vi "Configure Output Impedance.vi"(8 "error in (no error)":errorcluster, 10 "Impedance (0: 50 Ohms)":u16(ring) items=["50 Ohms", "High Impedance"], 11 "VISA resource name":refnum<visa-resource-name>) -> (0 "error out":errorcluster, 3 "VISA resource name out":refnum<visa-resource-name>)   [LabVIEW 2015, in "Template - Function Generator.lvlib"]
doc: "Configures the output impedance for the function generator."
uses:
  <instrlib>/_Template - Function Generator/Template - Function Generator.lvlib
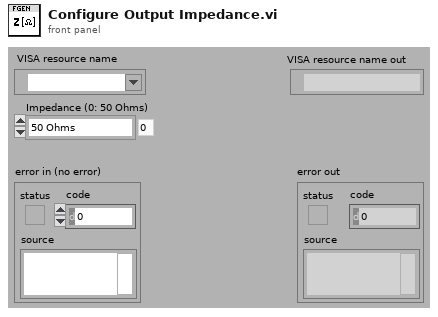
[diagram p1: front panel]
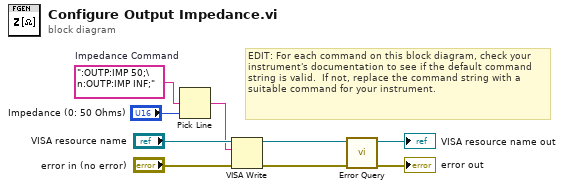
[diagram p0: block diagram]
diagram:
  w3 = ":OUTP:IMP 50;\n:OUTP:IMP INF;"  # Impedance Command
  # "EDIT: For each command on this block diagram, check your instrument's documentation to see if the default command string is valid.  If not, replace the command string with a suitable command for your instrument."
  n1 = Pick Line(multi-line string=w3, line index="Impedance (0: 50 Ohms)") -> (output string=w1:string)  [unwired: 1 in]
  n2 = VISA Write(VISA resource name="VISA resource name", write buffer=w1, error in (no error)="error in (no error)") -> (VISA resource name out=w5:refnum<visa-resource-name>, error out=w4:errorcluster)  [unwired: 1 out]
  n3 = call <instrlib>:"Error Query.vi"("error in (no error)"=w4, "VISA resource name"=w5) -> ("error out"=→"error out":errorcluster, "VISA resource name out"=→"VISA resource name out":refnum<visa-resource-name>)  [unwired: 6 in, 2 out]
